vi "New MCListbox Item Names Binding.vi"(9 "Set To Top Left?":T1, 10 "MCListbox Refnum":refnum<vi>) -> (0 "error out":errorcluster, 3 "MCListboxItemNamesBinding":refnum<class "MCListboxItemNamesBinding.lvclass">)   [LabVIEW 2017, in "Transport.lvlib" / "MCListboxItemNamesBinding.lvclass"]
doc: "<License>\nCopyright © 2017 Composed Systems, LLC | All rights reserved\nwww.composed.io\n\nAuthor: Ethan Stern <ethan.stern@composed.io>\n\nThis software is provided \"AS IS\" WITHOUT WARRANTIES, either express or implied, AND IS FOR EDUCATIONAL PURPOSES ONLY.\n</License>"
uses:
  MCListboxItemNamesBinding.lvclass
  MCListbox Binding Options.ctl
  MCListboxItemNamesBinding.lvclass/MCListboxItemNamesBinding.ctl
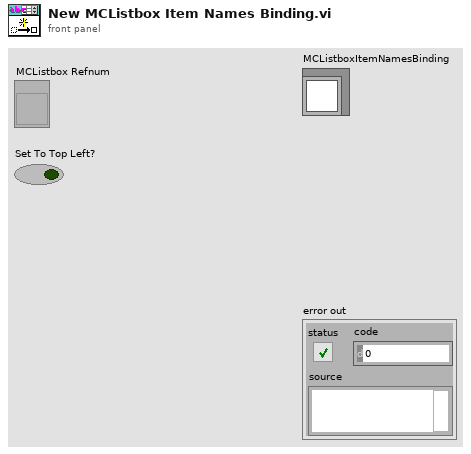
[diagram p1: front panel]
types:
  T1 = typedef "Transport.lvlib/MCListboxItemNamesBinding.lvclass/MCListbox Binding Options.ctl" = bool
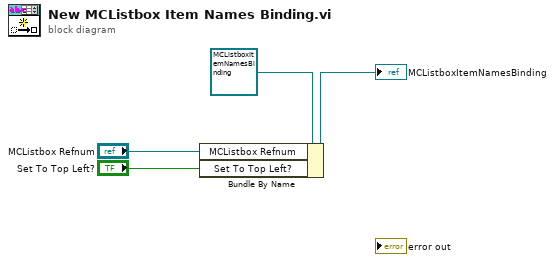
[diagram p0: block diagram]
diagram:
  n1 = Bundle By Name(cluster=refnum<class "MCListboxItemNamesBinding.lvclass"> refnum ("TerminalBinding in"), "MCListbox Refnum"="MCListbox Refnum", "Set To Top Left?"="Set To Top Left?") -> (→"MCListboxItemNamesBinding":refnum<class "MCListboxItemNamesBinding.lvclass">)
